vi "Initialize.vi"(6 "optional":variant, 8 "error in (no error)":errorcluster, 11 "LinkedList in":refnum<class "LinkedList.lvclass">) -> (0 "error out":errorcluster, 3 "LinkedList out":refnum<class "LinkedList.lvclass">)   [LabVIEW 2009, in "LinkedList.lvclass"]
uses:
  LinkedList.lvclass
  Structure/Structure.lvclass
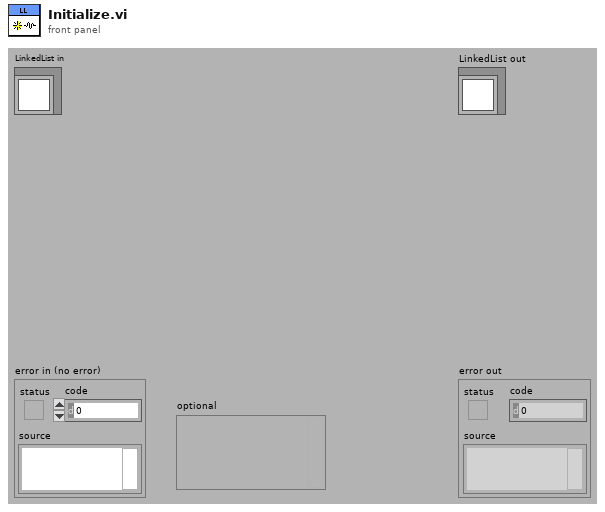
[diagram p1: front panel]
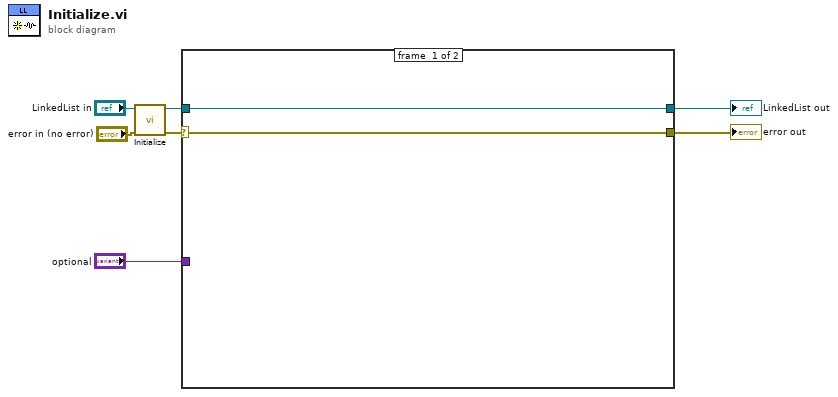
[diagram p0: block diagram]
diagram:
  n1 = call-parent "Initialize.vi"("error in (no error)"="error in (no error)", "Structure in"="LinkedList in") -> ("error out"=w3:errorcluster, "Structure out"=w1:refnum<class "LinkedList.lvclass">)  [unwired: 8 in]
  n2 = case shown="No Error" w3 {
    selector: w3 -> [w9 w11]
    tunnel: [w9 w11] -> w7
    tunnel: [w8 w10] -> w6
    tunnel: w1 -> [w8 w10]
    tunnel: "optional" -> [_ _]
    frame #0 {
    }
    frame #1 {
    }
  }
  "error out" <- w7
  "LinkedList out" <- w6
